vi "Getu32_array.vi"(8 "error in (no error)":errorcluster, 11 "OneOfTemplate in":refnum<class "nixnet_grpc_GetPropertyResponse_property_value.lvclass">) -> (0 "error out":errorcluster, 2 "Get_Val":T1, 3 "OneOfTemplate out":refnum<class "nixnet_grpc_GetPropertyResponse_property_value.lvclass">)   [LabVIEW 2019, in "grpc-xnet_client.lvlib" / "nixnet_grpc_GetPropertyResponse_property_value.lvclass"]
uses:
  nixnet_grpc_GetPropertyResponse_property_value.lvclass
  nixnet_grpc_U32Array.ctl
  nixnet_grpc_GetPropertyResponse_property_value.lvclass/nixnet_grpc_GetPropertyResponse_property_value.ctl
  grpc-xnet_client.lvlib
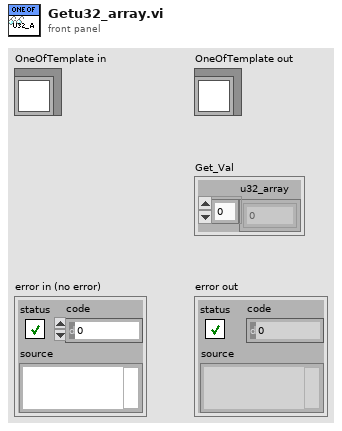
[diagram p1: front panel]
types:
  T1 = typedef "grpc-xnet_client.lvlib/nixnet_grpc_U32Array.ctl" = cluster{"u32_array":u32[]}
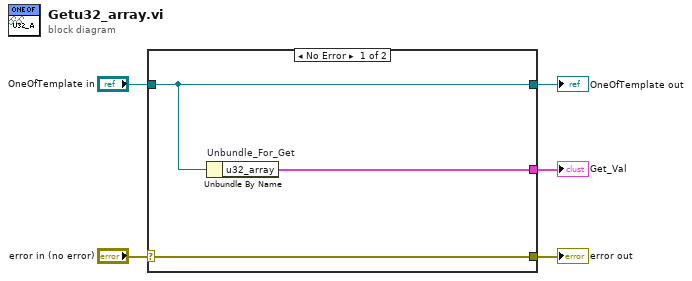
[diagram p0: block diagram]
diagram:
  n1 = case shown="No Error" "error in (no error)" {
    selector: "error in (no error)" -> [w8 w9]
    tunnel: [w8 w9] -> w4
    tunnel: [w7 w10] -> w2
    tunnel: "OneOfTemplate in" -> [w7 w10]
    tunnel: [w6 _] -> w1
    frame No Error {
      n2 = Unbundle By Name "Unbundle_For_Get"(w7) -> ("u32_array"=w6:T1)
    }
    frame Error {
    }
  }
  "error out" <- w4
  "OneOfTemplate out" <- w2
  "Get_Val" <- w1
